vi "Initiate.vi"(8 "Error In":errorcluster, 11 "Keithley 6482 In":refnum<visa-resource-name>) -> (0 "Error Out":errorcluster, 3 "Keithley 6482 Out":refnum<visa-resource-name>)   [LabVIEW 2009, in "Keithley-6482-Visa.lvlib"]
uses:
  <instrlib>/Keithley-6482-Visa9.0/Keithley-6482-Visa.lvlib
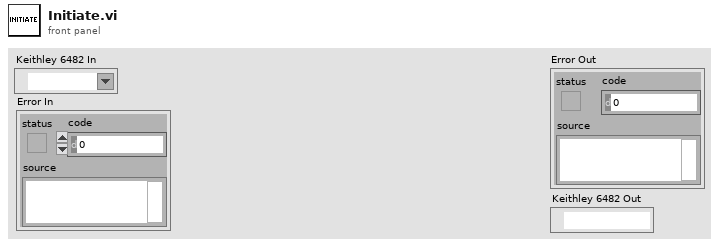
[diagram p1: front panel]
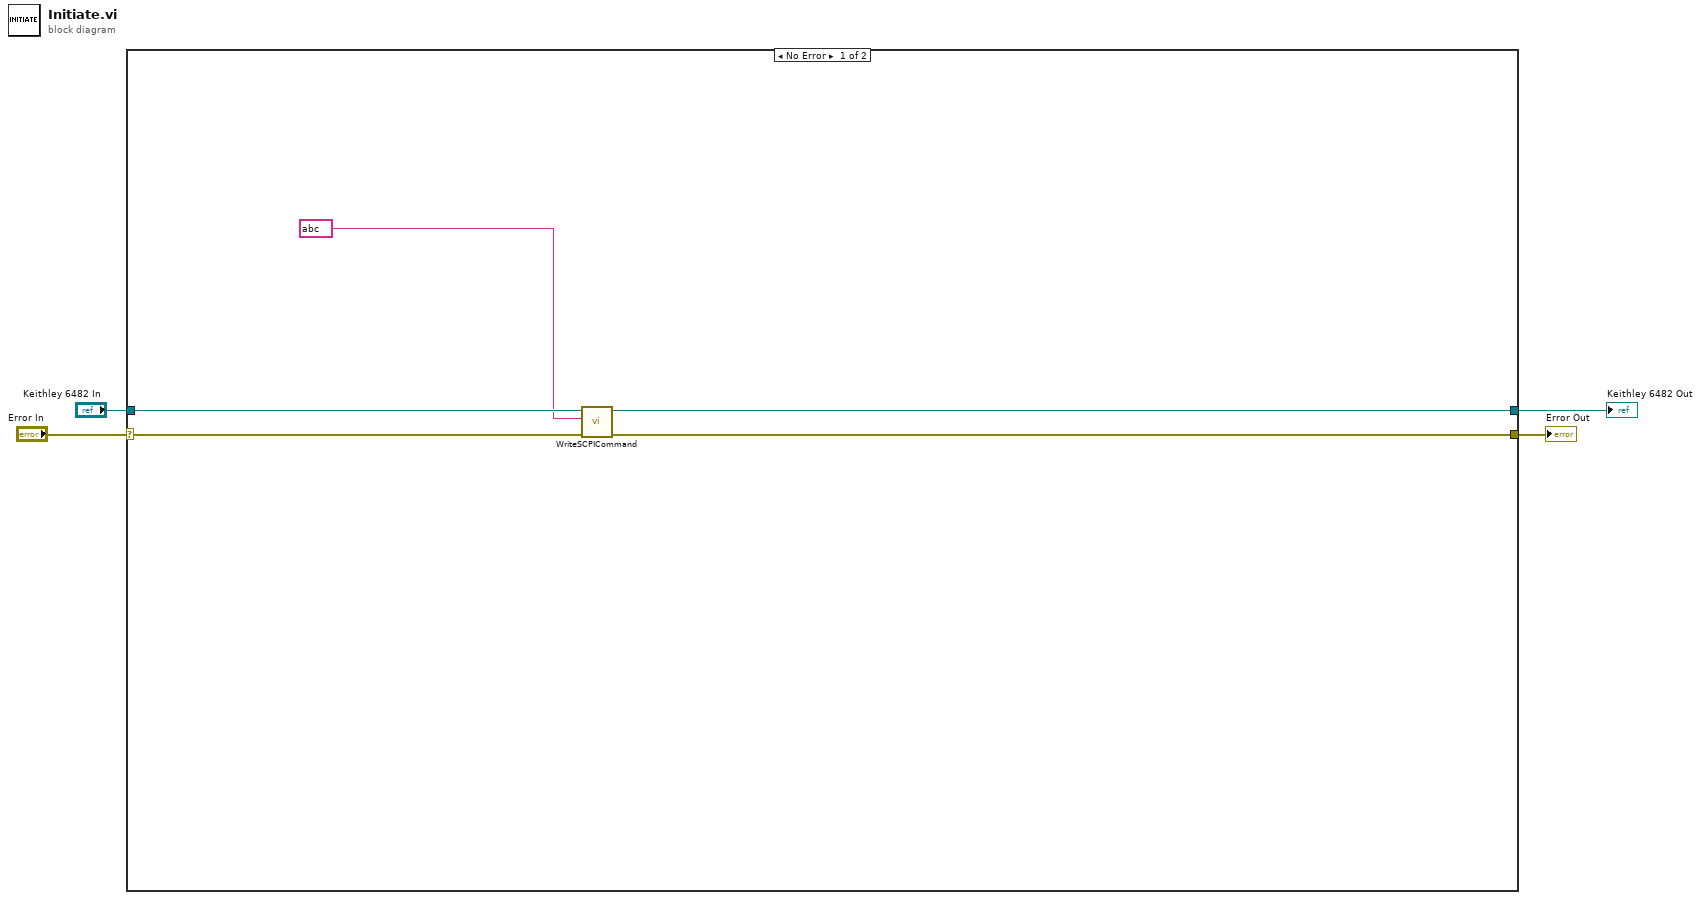
[diagram p0: block diagram]
diagram:
  n1 = case shown="No Error" "Error In" {
    selector: "Error In" -> [w9 w10]
    tunnel: "Keithley 6482 In" -> [w8 w11]
    tunnel: [w6 w10] -> w2
    tunnel: [w7 w11] -> w1
    frame #0 {
      n2 = call <instrlib>:"WriteSCPICommand.vi"("Error In"=w9, "SCPI Command"=string ? ("string"), "Keithley 6482 In"=w8) -> ("Error Out"=w6:errorcluster, "Keithley 6482 Out"=w7:refnum<visa-resource-name>)  [unwired: 7 in]
    }
    frame #1 {
    }
  }
  "Error Out" <- w2
  "Keithley 6482 Out" <- w1
